vi "Process.vi"(0 "Module Data In":T1, 11 "error in (no error)":errorcluster) -> (4 "Module Data Out":T1, 15 "error out":errorcluster)   [LabVIEW 2020, in "Template.lvlib"]
doc: "Initializes and run the processes in the Process Array one after the other."
uses:
  Template.lvlib
  Controls/Module - Data.ctl
  Modules.ctl
  Controls/Module - States.ctl
  Controls/Timing - Data.ctl
  Controls/Process - Element.ctl
  Controls/Process.ctl
  Controls/Process - Status.ctl
  Controls/Timing - Mode.ctl
  Controls/Message.ctl
  Error Handler - Logger Module/Error Handler - Logger.lvlib
panel:
  out "Process Status":string
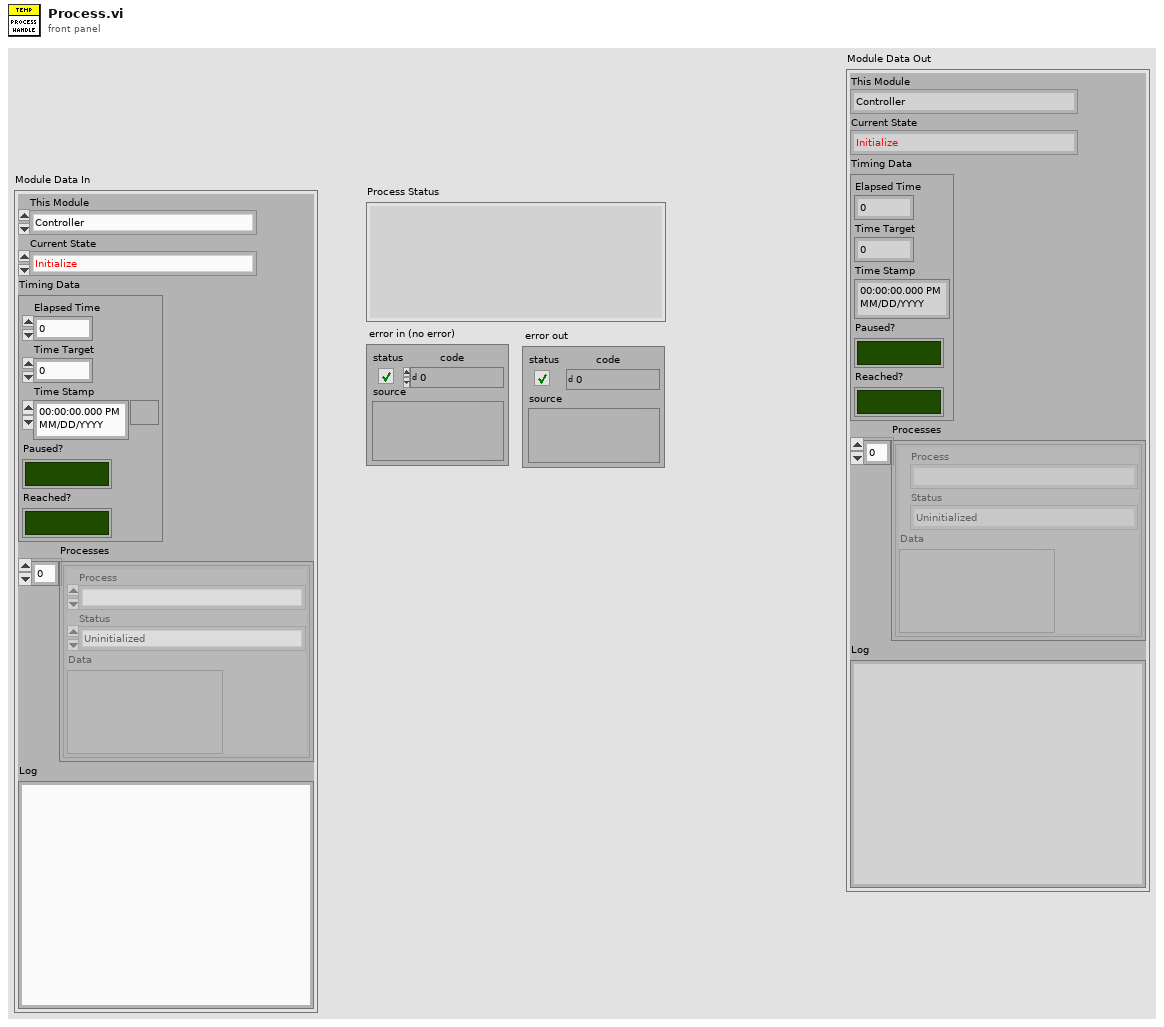
[diagram p1: front panel]
types:
  T1 = typedef "Template.lvlib/Module - Data.ctl" = cluster{"This Module":T2, "Current State":T3, "Timing Data":T4, "Processes":T5[], "Log":string}
  T2 = typedef "Error Handler - Logger.lvlib/Modules.ctl" = enum16{"Controller", "Error Handler - Logger"}
  T3 = typedef "Template.lvlib/Module - States.ctl" = enum16{"Initialize", "Event ", "Send data", "FP Element: Update", "FP Element: Disable/Enable", "Timer: Setup", "Terminate", "---------------Template---------------"}
  T4 = typedef "Template.lvlib/Timing - Data.ctl" = cluster{"Elapsed Time":dbl, "Time Target":dbl, "Time Stamp":timestamp, "Paused?":bool, "Reached?":bool}
  T5 = typedef "Template.lvlib/Process - Element.ctl" = cluster{"Process":T6, "Status":T7, "Data":variant}
  T6 = typedef "Template.lvlib/Process.ctl" = enum16{""}
  T7 = typedef "Template.lvlib/Process - Status.ctl" = enum16{"Uninitialized", "Busy"}
  T8 = typedef "Template.lvlib/Timing - Mode.ctl" = enum16{"Reset", "Read", "Pause", "Resume"}
  T9 = typedef "Template.lvlib/Message.ctl" = cluster{"State":T3, "Data":variant, "Transitioning State?":bool}
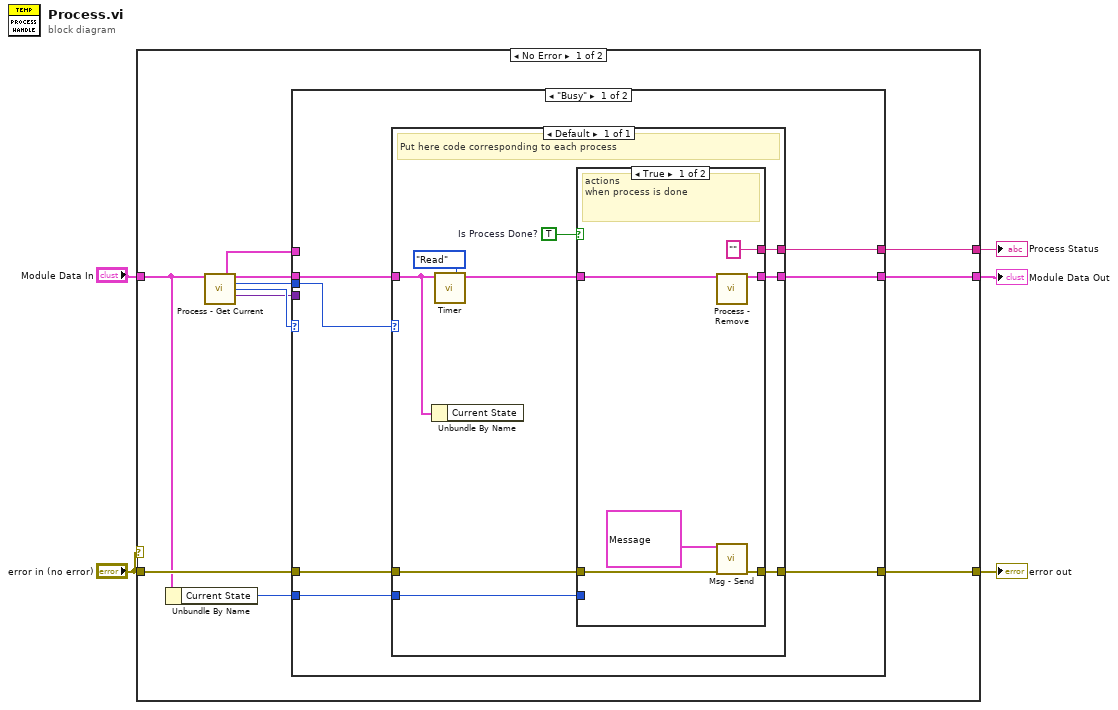
[diagram p0: block diagram]
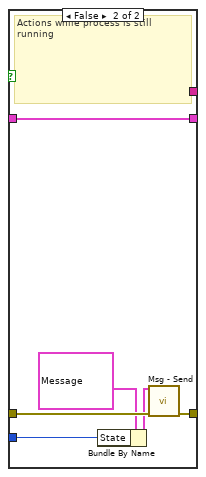
[diagram p2: hidden frame]
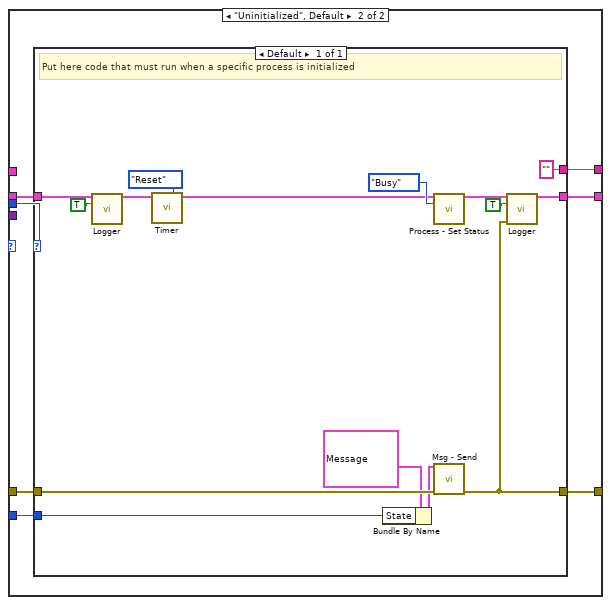
[diagram p3: hidden frame]
diagram:
  n1 = case shown="No Error" "error in (no error)" {
    tunnel: [w16 w68] -> w5
    tunnel: "Module Data In" -> [w8 w68]
    tunnel: [w14 w67] -> w3
    tunnel: "error in (no error)" -> [w9 w67]
    tunnel: [w6 _] -> w1
    frame No Error {
      n2 = Unbundle By Name(w8) -> ("Current State"=w7:T3)
      n3 = call "Process - Get Current.vi"("Module Data In"=w8) -> ("|Current Process"=w10:T5, "Module Data Out"=w15:T1, "Process"=w13:T6, "Status"=w12:T7, "Data"=w11:variant)  [unwired: 9 in, 1 out]
      n4 = case shown="\"Busy\"" w12 {
        tunnel: [w22 w50] -> w16
        tunnel: w15 -> [w23 w51]
        tunnel: [w19 w47] -> w14
        tunnel: w9 -> [w21 w49]
        tunnel: w13 -> [w20 w48]
        tunnel: w11 -> [_ _]
        tunnel: w10 -> [_ _]
        tunnel: w7 -> [w18 w46]
        tunnel: [w17 w45] -> w6
        frame "Busy" {
          n5 = case shown="Default" w20 {
            tunnel: [w32] -> w22
            tunnel: w23 -> [w26]
            tunnel: [w30] -> w19
            tunnel: w21 -> [w31]
            tunnel: w18 -> [w25]
            tunnel: [w24] -> w17
            frame Default {
              w29 = TRUE  # Is Process Done?
              # "Put here code corresponding to each process"
              n6 = Unbundle By Name(w26) -> ()  [unwired: 1 out]
              n7 = call "Timer.vi"("Mode"=Timing_-_Mode."Read", "Module Data In"=w26) -> ("Module Data Out"=w28:T1)  [unwired: 6 in, 3 out]
              n8 = case shown="True" w29 {
                tunnel: [w37 w44] -> w32
                tunnel: w28 -> [w38 w44]
                tunnel: [w36 w43] -> w30
                tunnel: w31 -> [w35 w42]
                tunnel: w25 -> [_ w41]
                tunnel: ["" ("Process Status") _] -> w24
                frame True {
                  # "actions\nwhen process is done"
                  n9 = call "Process - Remove.vi"("Module Data In"=w38) -> ("Module Data Out"=w37:T1)  [unwired: 13 in, 1 out]
                  n10 = call "Msg - Send.vi"("Message"=T9 {"State"=enum."Initialize", "Data"=variant, "Transitioning State?"=TRUE}, "error in (no error)"=w35) -> ("error out"=w36:errorcluster)  [unwired: 13 in]
                }
                frame False {
                  # "Actions while process is still running"
                  n11 = Bundle By Name(cluster=T9 {"State"=enum."Initialize", "Data"=variant, "Transitioning State?"=FALSE} ("Message"), "State"=w41) -> (w39:T9)
                  n12 = call "Msg - Send.vi"("Message"=w39, "error in (no error)"=w42) -> ("error out"=w43:errorcluster)  [unwired: 13 in]
                }
              }
            }
          }
        }
        frame "Uninitialized", Default {
          n13 = case shown="Default" w48 {
            tunnel: [w57] -> w50
            tunnel: w51 -> [w54]
            tunnel: [w52] -> w47
            tunnel: w49 -> [w66]
            tunnel: w46 -> [w64]
            tunnel: ["" ("Process Status")] -> w45
            frame Default {
              # "Put here code that must run when a specific process is initialized"
              n14 = call "Logger.vi"("Module Data In"=w54, "Log Process?"=TRUE) -> ("Module Data Out"=w53:T1)  [unwired: 12 in, 1 out]
              n15 = call "Timer.vi"("Mode"=Timing_-_Mode."Reset", "Module Data In"=w53) -> ("Module Data Out"=w56:T1)  [unwired: 6 in, 3 out]
              n16 = Bundle By Name(cluster=T9 {"State"=enum."Initialize", "Data"=variant, "Transitioning State?"=FALSE} ("Message"), "State"=w64) -> (w62:T9)
              n17 = call "Process - Set Status.vi"("Module Data In"=w56, "Status"=Process_-_Status."Busy") -> ("Module Data Out"=w58:T1)  [unwired: 12 in, 1 out]
              n18 = call "Msg - Send.vi"("Message"=w62, "error in (no error)"=w66) -> ("error out"=w52:errorcluster)  [unwired: 13 in]
              n19 = call "Logger.vi"("Module Data In"=w58, "Log Process?"=TRUE, "error in (no error)"=w52) -> ("Module Data Out"=w57:T1)  [unwired: 11 in, 1 out]
            }
          }
        }
      }
    }
    frame Error {
    }
  }
  "error out" <- w3
  "Module Data Out" <- w5
  "Process Status" <- w1
